vi "Add Global Path Args Handler.vi"(11 "Controller Handler Map In":T1) -> (3 "Controller Handler Map":T1)   [LabVIEW 2020, in "HTTP Server.lvlib" / "Server.lvclass"]
uses:
  Server.lvclass
  Controller Handler Map.ctl
  Priority.ctl
  Controller Handler/Controller Handler.lvclass
  ControllerIndexedPathParams Handler/ControllerIndexedPathParams Handler.lvclass
  C:/dev/lv20CE/relink/lv-http-server/HTTP Server/Controller Handler/Controller Handler.lvclass
  HTTP Server.lvlib
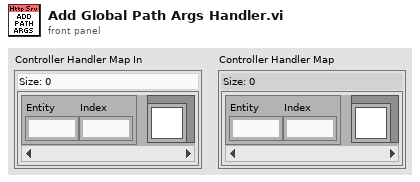
[diagram p1: front panel]
types:
  T1 = typedef "HTTP Server.lvlib/Controller Handler Map.ctl" = map{T2, refnum<class "Controller Handler.lvclass">}
  T2 = typedef "HTTP Server.lvlib/Priority.ctl" = cluster{"Entity":u16, "Index":u16}
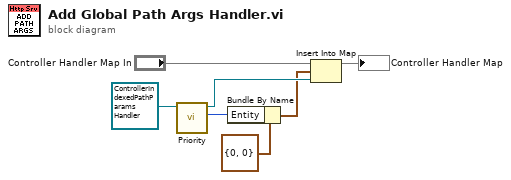
[diagram p0: block diagram]
diagram:
  n1 = call-dynamic "Priority.vi"("Handler in"=refnum<class "ControllerIndexedPathParams Handler.lvclass"> refnum ("HTTP Server.lvlib:ControllerIndexedPathParams Handler.lvclass")) -> ("Priority"=w4:u16, "Handler out"=w2:refnum<class "ControllerIndexedPathParams Handler.lvclass">)  [unwired: 8 in, 1 out]
  n2 = Bundle By Name(cluster=T2 {"Entity"=0, "Index"=0} ("Priority"), "Entity"=w4) -> (w1:T2)
  n3 = Insert Into Map(map in="Controller Handler Map In", key=w1, value=w2) -> (map out=→"Controller Handler Map":T1)  [unwired: 2 out]
